vi "Load Flattened 32bit float Image from Tiff.vi"(0 "path to TIFF file":path=path "/HD1/Users/herbertlooser/Desktop/Ladungsspr焗er.tif", 1 "error in (no error)":errorcluster) -> (5 "Gray16/32":sgl[][](array[numeric]), 7 "error out":errorcluster)   [LabVIEW 2015, in "Tiff reader.lvlib"]
doc: "This .vi is taken from an online tiff reader. It is able to read 32-bit floating point .tiff images."
uses:
  Tiff reader.lvlib
panel:
  out "Intensity Graph":sgl[][](graph)
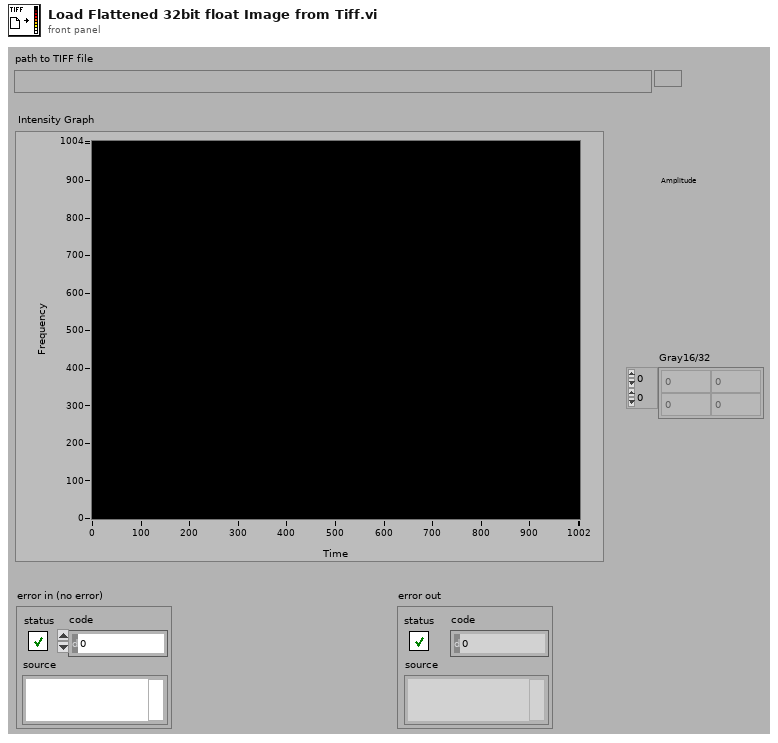
[diagram p1: front panel]
types:
  T1 = enum16{"open", "open or create", "create or replace", "create"}
  T2 = typedef "Tiff reader.lvlib/IFD Entry.ctl" = cluster{"Tag":u16, "Type":T3, "Count":u32, "Val/Offs":u32, "Is Pointer?":bool, "Byte stream index":i32}
  T3 = typedef "Tiff reader.lvlib/FieldTypes.ctl" = enum16{"NULL", "U8", "ASCII7", "U16", "U32", "RATIONAL", "SByte(I8)", "Undef(8Bit)", "I16", "I32", "SRat(4B:4B)", "SGL(4Byte)", "DBL(8Byte)"}
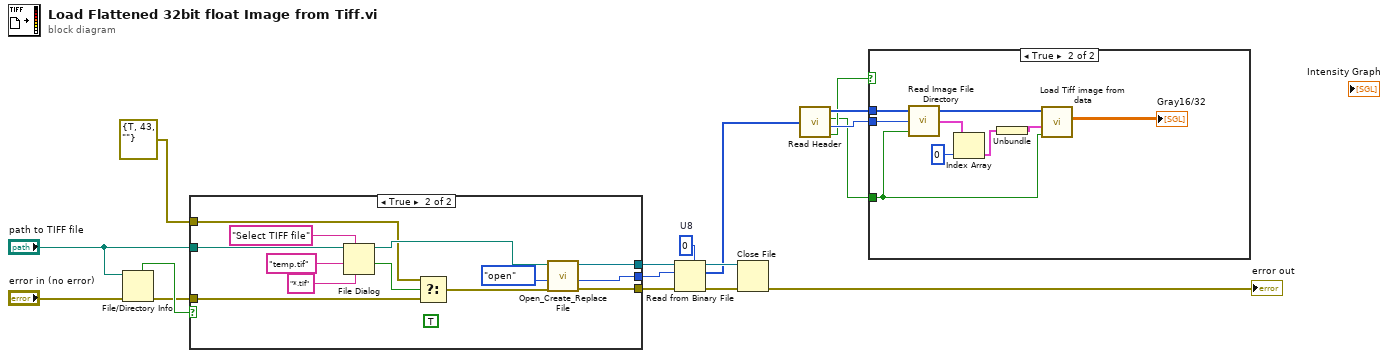
[diagram p0: block diagram]
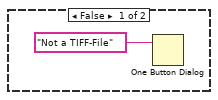
[diagram p2: hidden frame]
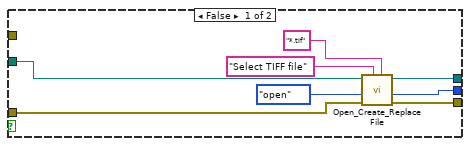
[diagram p3: hidden frame]
diagram:
  w2 = u8 0  # U8
  n1 = File/Directory Info(path="path to TIFF file", error in="error in (no error)") -> (directory=w12:bool, error out=w3:errorcluster)  [unwired: 5 out]
  n2 = case shown="True" w12 {
    tunnel: [w22 w31] -> w17
    tunnel: [w21 w33] -> w16
    tunnel: [w20 w32] -> w13
    tunnel: w3 -> [w19 w29]
    tunnel: "path to TIFF file" -> [w18 w26]
    tunnel: errorcluster {"status"=TRUE, "code"=43, "source"=""} ("error in (no error)") -> [_ w27]
    frame False {
      n3 = call <vilib>:"Open_Create_Replace File.vi"("pattern"="*.tif", "prompt"="Select TIFF file", "error in (no error)"=w19, "function (open:0)"=T1."open", "file path"=w18) -> ("error out"=w20:errorcluster, "file size (bytes)"=w22:i32, "refnum"=w21:refnum<file>)  [unwired: 2 in, 2 out]
    }
    frame True {
      (unwired) TRUE ("advisory dialog? (display:T)")
      n4 = File Dialog(6:"*.tif" ("pattern"), 7:"Select TIFF file" ("prompt"), 9:"temp.tif" ("default name"), 11:w26) -> (1:w30:bool, 3:w35:path)  [unwired: 1 in, 4 out]
      n5 = Select(t=w27, s=w30, f=w29) -> (s? t:f=w28:errorcluster)
      n6 = call <vilib>:"Open_Create_Replace File.vi"("error in (no error)"=w28, "function (open:0)"=T1."open", "file path"=w35) -> ("error out"=w32:errorcluster, "file size (bytes)"=w31:i32, "refnum"=w33:refnum<file>)  [unwired: 3 in, 3 out]
    }
  }
  n7 = Read from Binary File(5:w2, 8:w13, 10:w17, 11:w16) -> (0:w14:errorcluster, 2:w1:u8[], 3:w15:refnum<file>)  [unwired: 3 out]
  n8 = Close File(refnum=w15, error in=w14) -> (error out=→"error out":errorcluster)  [unwired: 1 out]
  n9 = call "Read Header.vi"("TIFF Data in"=w1) -> ("TIFF Data out"=w9:u8[], "Litt/BigEnd"=w6:bool, "ImFileDirectOffs"=w8:u32, "IsTIFF?"=w7:bool)
  n10 = case shown="True" w7 {
    tunnel: w9 -> [_ w48]
    tunnel: w8 -> [_ w47]
    tunnel: w6 -> [_ w45]
    frame False {
      n11 = One Button Dialog(message="Not a TIFF-File") -> ()  [unwired: 2 out]
    }
    frame True {
      n12 = call "Read Image File Directory.vi"("Litt/BigEnd"=w45, "Im_File_Dir Offs"=w47, "Image Data in"=w48) -> ("Directories"=w44:cluster{"Tags":T2[]}[], "Image Data out"=w46:u8[])  [unwired: 1 out]
      n13 = Index Array(array=w44, index=0 ("index (row)")) -> (element=w41:cluster{"Tags":T2[]})
      n14 = Unbundle(w41) -> ("Tags"=w40:T2[])
      n15 = call "Load Tiff image from data.vi"("Litt/BigEnd"=w45, "DirEntries"=w40, "Image Data in"=w46) -> ("Gray16/32"=→"Gray16/32":sgl[][])  [unwired: 8 out]
    }
  }
